vi "Finish Flatten VI.vi"(7 "BD":refnum<vi>, 8 "error in (no error)":errorcluster, 10 "Prev Term":refnum<vi>, 11 "LV-Protoc in":refnum<class "LV-Protoc.lvclass">) -> (0 "error out":errorcluster, 3 "LV-Protoc out":refnum<class "LV-Protoc.lvclass">)   [LabVIEW 2020, in "LV-Protoc.lvlib" / "LV-Protoc.lvclass"]
uses:
  LV-Protoc.lvclass
  <vilib>/Utility/traverseref.llb/TRef TravTarget.ctl
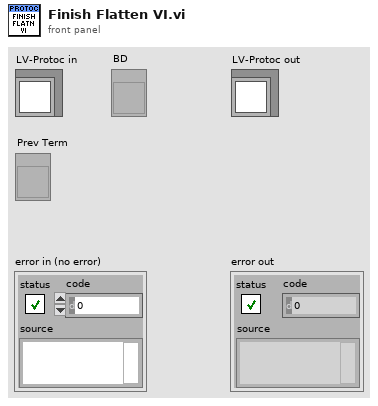
[diagram p1: front panel]
types:
  T1 = typedef "TRef TravTarget.ctl" = enum16{"FP", "BD", "Other"}
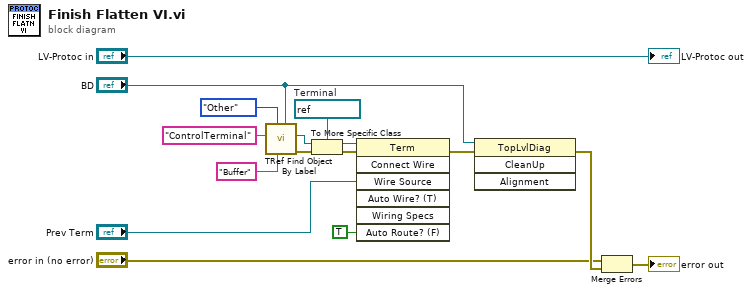
[diagram p0: block diagram]
diagram:
  w16 = refnum<vi> refnum  # Terminal
  n1 = call <vilib>:"TRef Find Object By Label.vi"("Other Refnum"="BD", "Label"="Buffer", "Traverse Target"=TRef_TravTarget."Other", "Class Name"="ControlTerminal") -> ("error out"=w15:errorcluster, "Found Obj Ref"=w14:refnum<vi>)  [unwired: 4 in, 2 out]
  n2 = To More Specific Class(target class=w16, reference=w14, error in=w15) -> (specific class reference=w10:refnum<vi>, error out=w9:errorcluster)
  n3 = invoke class="Term" method="Connect Wire"(reference=w10, error in=w9, "Wire Source"="Prev Term", "Auto Route? (F)"=TRUE) -> (error out=w6:errorcluster)  [unwired: 3 in, 6 out]
  n4 = invoke class="TopLvlDiag" method="CleanUp"(reference="BD", error in=w6) -> (error out=w4:errorcluster)  [unwired: 2 in, 3 out]
  n5 = Merge Errors("error in (no error)", w4) -> (→"error out":errorcluster)
  "LV-Protoc out" <- "LV-Protoc in"
